vi "PH_GUI.set string GUI object.vi"(1 "Visible (True)":bool=TRUE, 2 "GUI object Ref":refnum<vi>, 3 "Text":string, 4 "Blinking? (false)":bool, 5 "error in":errorcluster caption="error in (no error)", 7 "Caption (N/A)":string="N/A") -> (19 "error out":errorcluster)   [LabVIEW 2014, in "PH_Common.lvlib"]
doc: "Sets value and more for the referenced GUI object."
uses:
  PH_Common.lvlib
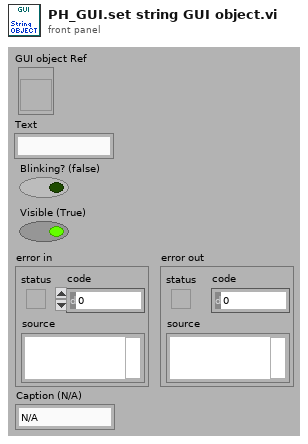
[diagram p1: front panel]
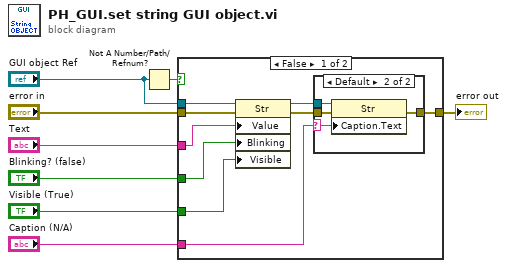
[diagram p0: block diagram]
diagram:
  n1 = Not A Number/Path/Refnum?(number/path/refnum="GUI object Ref") -> (NaN/Path/Refnum?=w5:bool)
  n2 = case shown="False" w5 {
    tunnel: "GUI object Ref" -> [w16 _]
    tunnel: "error in" -> [w17 w23]
    tunnel: [w11 w23] -> w7
    tunnel: "Text" -> [w15 _]
    tunnel: "Blinking? (false)" -> [w14 _]
    tunnel: "Visible (True)" -> [w13 _]
    tunnel: "Caption (N/A)" -> [w9 _]
    frame False {
      n3 = property class="Str"(reference=w16, error in=w17, "Value"=w15, "Blinking"=w14, "Visible"=w13) -> (reference out=w10:refnum<vi>, error out=w12:errorcluster)
      n4 = case shown="Default" w9 {
        selector: w9 -> [_ w19]
        tunnel: w12 -> [w18 w22]
        tunnel: [w18 w21] -> w11
        tunnel: w10 -> [_ w20]
        frame "", "N/A" {
        }
        frame Default {
          n5 = property class="Str"(reference=w20, error in=w22, "Caption.Text"=w19) -> (error out=w21:errorcluster)  [unwired: 1 out]
        }
      }
    }
    frame True {
    }
  }
  "error out" <- w7
